vi "Set Frequency.vi"(8 "error in (no error)":errorcluster, 10 "test signal freq":dbl[unit], 11 "VISA resource name":refnum<visa-resource-name>) -> (0 "error out":errorcluster, 3 "VISA resource name out":refnum<visa-resource-name>)   [LabVIEW 2017]
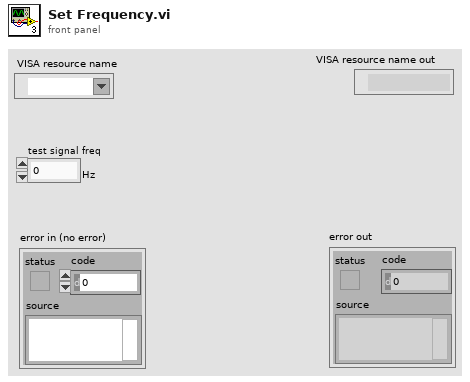
[diagram p1: front panel]
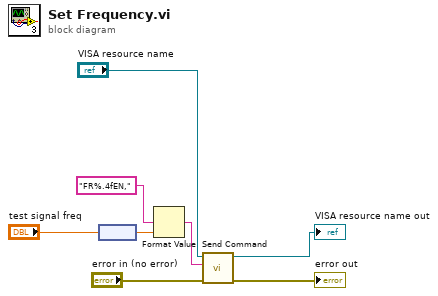
[diagram p0: block diagram]
diagram:
  n1 = node("test signal freq") -> (w1:dbl)
  n2 = Format Value(format string="FR%.4fEN,", value (0)=w1) -> (output string=w8:string)  [unwired: 1 in]
  n3 = call "Send Command.vi"("error in (no error)"="error in (no error)", "write buffer"=w8, "VISA resource name"="VISA resource name") -> ("error out"=→"error out":errorcluster, "VISA resource name out"=→"VISA resource name out":refnum<visa-resource-name>)  [unwired: 7 in]
